vi "Toggle Digital Increment Decrement Visible ( Swithc Show Or Hide ).vi"(6 "Variant in":variant, 7 "Shift Pressed?":bool, 8 "error in (no error)":errorcluster, 10 "QD Combo Box Ref":refnum<vi>, 11 "QD Launch VI Ref":refnum<vi>) -> (0 "error out":errorcluster, 4 "Variant out":variant)   [LabVIEW 2020, in "Control Operation.lvlib"]
doc: "Toggle Digital Increment Decrement Visible ( Swithc Show Or Hide ).vi"
uses:
  Control Operation.lvlib
panel:
  in  "Undo Name":string="Toggle Digital Increment Decrement Visible ( Swithc Show Or Hide ).vi"
  # "Do not change the connector pane of this VI.\n\nSee the block diagram for directions on how to use this template."
  # "Specify the name of the Undo transaction"
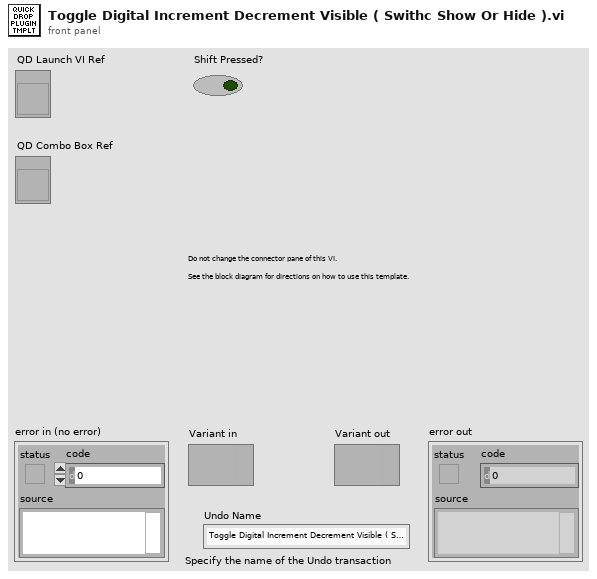
[diagram p1: front panel]
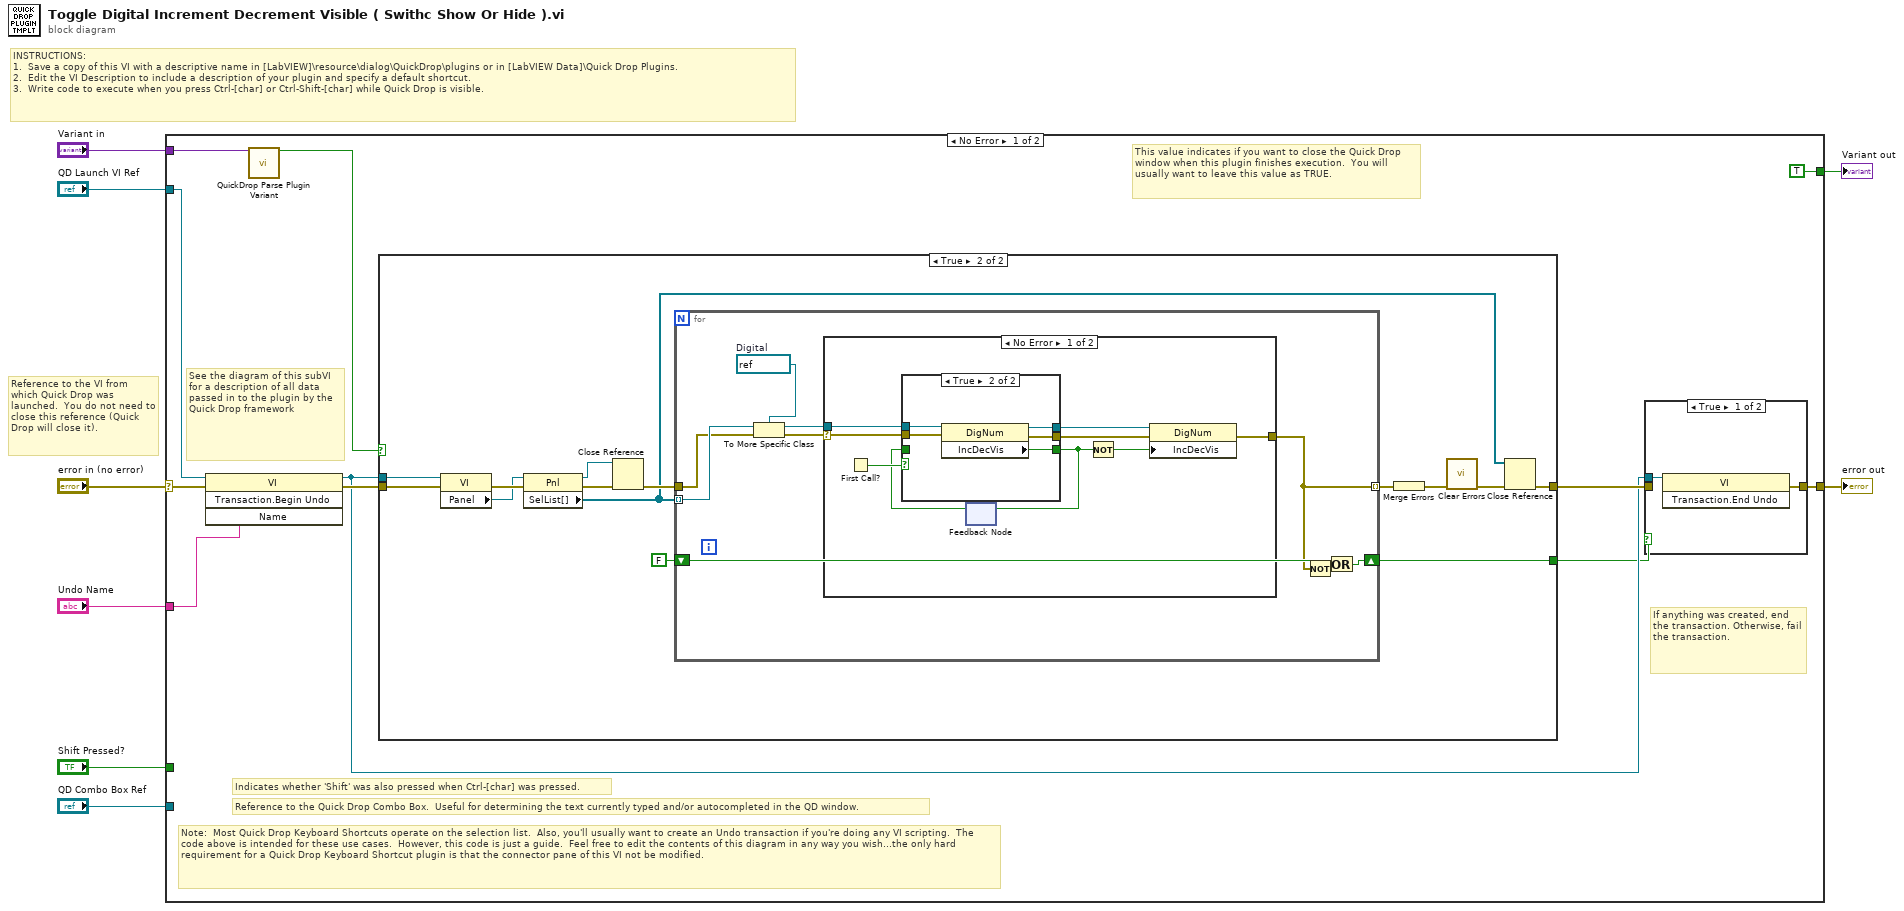
[diagram p0: block diagram]
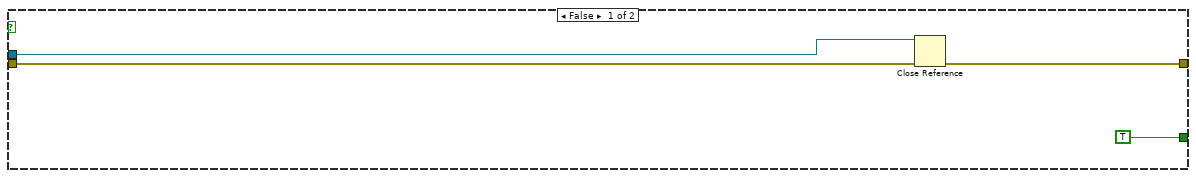
[diagram p2: hidden frame]
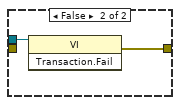
[diagram p5: hidden frame]
diagram:
  # "Reference to the VI from which Quick Drop was launched.  You do not need to close this reference (Quick Drop will close it)."
  # "INSTRUCTIONS:\n1.  Save a copy of this VI with a descriptive name in [LabVIEW]\\resource\\dialog\\QuickDrop\\plugins or in [LabVIEW Data]\\Quick Drop Plugins.\n2.  Edit the VI Description to include a description of your plugin and specify a default shortcut. \n3.  Write code to execute when you press Ctrl-[char] or Ctrl-Shift-[char] while Quick Drop is visible."
  n1 = case shown="No Error" "error in (no error)" {
    selector: "error in (no error)" -> [w18 w69]
    tunnel: [w12 w69] -> w7
    tunnel: "QD Launch VI Ref" -> [w17 _]
    tunnel: "Shift Pressed?" -> [_ _]
    tunnel: "QD Combo Box Ref" -> [_ _]
    tunnel: "Variant in" -> [w19 _]
    tunnel: "Undo Name" -> [w16 _]
    tunnel: [TRUE _] -> w1
    frame No Error {
      # "Note:  Most Quick Drop Keyboard Shortcuts operate on the selection list.  Also, you'll usually want to create an Undo transaction if you're doing any VI scripting.  The code above is intended for these use cases.  However, this code is just a guide.  Feel free to edit the contents of this diagram in any way you wish...the only hard requirement for a Quick Drop Keyboard Shortcut plugin is that the connector pane of this VI not be modified."
      # "If anything was created, end the transaction. Otherwise, fail the transaction."
      # "This value indicates if you want to close the Quick Drop window when this plugin finishes execution.  You will usually want to leave this value as TRUE."
      # "See the diagram of this subVI for a description of all data passed in to the plugin by the Quick Drop framework"
      # "Reference to the Quick Drop Combo Box.  Useful for determining the text currently typed and/or autocompleted in the QD window."
      # "Indicates whether 'Shift' was also pressed when Ctrl-[char] was pressed."
      n2 = invoke class="VI" method="Transaction.Begin Undo"(reference=w17, error in=w18, "Name"=w16) -> (reference out=w10:refnum<vi>, error out=w13:errorcluster)  [unwired: 1 in, 2 out]
      n3 = call <vilib>:"QuickDrop Parse Plugin Variant.vi"("QDKS Variant in"=w19) -> ("QD Launch VI Panel?"=w14:bool)  [unwired: 12 in, 2 out]
      n4 = case shown="True" w14 {
        tunnel: w13 -> [w22 w37]
        tunnel: [w21 w27] -> w11
        tunnel: w10 -> [w20 w35]
        tunnel: [TRUE w33] -> w9
        frame False {
          n5 = Close Reference(reference=w20, error in (no error)=w22) -> (error out=w21:errorcluster)
        }
        frame True {
          n6 = property class="VI"(reference=w35, error in=w37) -> (error out=w32:errorcluster, "Panel"=w31:refnum<vi>)  [unwired: 1 out]
          n7 = property class="Pnl"(reference=w31, error in=w32) -> (reference out=w29:refnum<vi>, error out=w30:errorcluster, "SelList[]"=w26:refnum<vi>[])
          n8 = Close Reference(reference=w29, error in (no error)=w30) -> (error out=w36:errorcluster)
          n9 = for {
            shift-right: [w45] -> w33
            shift-left: FALSE -> [w46]
            tunnel: w26 -> [w44] mode=indexing
            tunnel: w36 -> [w43]
            tunnel: [w40] -> w28 mode=indexing
            w38 = refnum<vi> refnum  # Digital
            n10 = To More Specific Class(target class=w38, reference=w44, error in=w43) -> (specific class reference=w42:refnum<vi>, error out=w41:errorcluster)
            n11 = case shown="No Error" w41 {
              selector: w41 -> [w54 w64]
              tunnel: w42 -> [w55 _]
              tunnel: [w51 w64] -> w40
              frame No Error {
                n12 = First Call?() -> (First Call?: T/F=w49:bool)
                n13 = feedback #1() -> (w47:bool)  [unwired: 1 in]
                n14 = case shown="True" w49 {
                  tunnel: w55 -> [w58 w63]
                  tunnel: w54 -> [w57 w62]
                  tunnel: [w58 w61] -> w53
                  tunnel: [w57 w60] -> w52
                  tunnel: [w56 w59] -> w48
                  tunnel: w47 -> [w56 _]
                  frame False {
                  }
                  frame True {
                    n15 = property class="DigNum"(reference=w63, error in=w62) -> (reference out=w61:refnum<vi>, error out=w60:errorcluster, "IncDecVis"=w59:bool)
                  }
                }
                n16 = feedback-in #1(w48) -> ()
                n17 = Not(x=w48) -> (.not. x?=w50:bool)
                n18 = property class="DigNum"(reference=w53, error in=w52, "IncDecVis"=w50) -> (error out=w51:errorcluster)  [unwired: 1 out]
              }
              frame Error {
              }
            }
            n19 = Not(x=w40) -> (.not. x?=w39:bool)
            n20 = Or(x=w46, y=w39) -> (x .or. y?=w45:bool)
          }
          n21 = Merge Errors(w28) -> (w25:errorcluster)
          n22 = call <vilib>:"Clear Errors.vi"("error in (no error)"=w25) -> ("error out"=w24:errorcluster)  [unwired: 5 in, 1 out]
          n23 = Close Reference(reference=w26, error in (no error)=w24) -> (error out=w27:errorcluster)
        }
      }
      n24 = case shown="True" w9 {
        tunnel: w10 -> [w65 w67]
        tunnel: [w66 w68] -> w12
        tunnel: w11 -> [_ _]
        frame True {
          n25 = invoke class="VI" method="Transaction.End Undo"(reference=w65) -> (error out=w66:errorcluster)  [unwired: 2 in, 2 out]
        }
        frame False {
          n26 = invoke class="VI" method="Transaction.Fail"(reference=w67) -> (error out=w68:errorcluster)  [unwired: 2 in, 2 out]
        }
      }
    }
    frame Error {
    }
  }
  "error out" <- w7
  "Variant out" <- w1
